vi "ReadWriteTest (host).vi"() -> ()   [LabVIEW 2012]
uses:
  <vilib>/rvi/interface/nirviOpenFPGA/nirviOpenFPGA.xnode
  ReadWriteTest (FPGA).vi
  <vilib>/rvi/interface/nirviReadWriteControl/nirviReadWriteControl.xnode
  <vilib>/rvi/interface/RandomDataEmulation/nirviRandomDataOpen.vi
panel:
  out "Point Read":cluster{"X":i32, "Y":i32, "Z":i32}
  out "Point Written":cluster{"X":i32, "Y":i32, "Z":i32}
  out "Read Time":u32
  out "Write Time":u32
  out "Count":i32
  out "Matched":cluster{"X":bool, "Y":bool, "Z":bool}
  in  "stop":bool
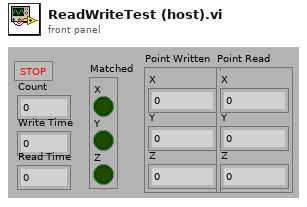
[diagram p1: front panel]
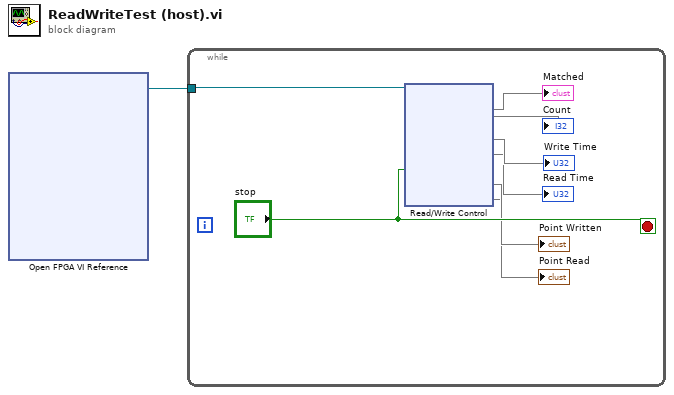
[diagram p0: block diagram]
diagram:
  n1 = xnode "Open FPGA VI Reference"() -> ("FPGA VI Reference Out"=w1:refnum<k20>)  [unwired: 2 in, 1 out]
  n2 = while {
    tunnel: w1 -> [w9]
    stop <- "stop" stop-if-true
    n3 = xnode "Read/Write Control"("FPGA VI Reference In"=w9, "stop"="stop") -> ("Matched"=→"Matched", "Numeric"=→"Count", "Write Time"=→"Write Time", "Read Time"=→"Read Time", "Point Written"=→"Point Written", "Point Read"=→"Point Read")  [unwired: 1 in, 2 out]
  }
